vi "MarkedRobot2ndStriker.vi"(6 "atacando ao contrário?":bool=TRUE, 8 "Função":T1, 9 "id":u32, 10 "IA State Input":T3={"our_robots"=[], "enemy_robots"=[], "balls"=[], "geometry"={"line_width"=0, "field_length"=0, "field_width"=0, "boundary_width"=0, "referee_width"=0, "goal_width"=0, "goal_depth"=0, "goal_wall_width"=0, "center_circle_radius"=0, "defense_radius"=0, "defense_stretch"=0, "free_kick_from_defense_dist"=0, "penalty_spot_from_field_line_dist"=0, "penalty_line_from_spot_dist"=0}, "IA Judge"={"stage"="", "command"="", "our_goalie_id"=0.0, "enemy_goalie_id"=0.0, "command enum"=enum."Halt", "Time"=enum."Azul"}, "Received Timestamp"=timestamp(0 s since 1904-01-01), "Events"={"Touch"=FALSE, "Ball out"=FALSE, "id touch"=0.0, "Ball out of \nVision"=FALSE, "Ball inside \nGoalie area"=FALSE, "Robot not responding"=FALSE, "Robots responding status"=[1.0, 1.0, 1.0, 1.0, 1.0, 1.0], "Enemy Ball \nPossession"=FALSE, "Pass State"=FALSE, "id end of pass"=0.0, "Kick"=FALSE, "Id ini Possession"=0.0, "Ball Possesion"=FALSE, "Id Possesion"=0.0, "Direct Kick"=FALSE, "2nd Strk Ativo"=FALSE}}, 11 "AI Parameters":T2={"GotoKick"={"Dist do cone a frente"=150.0, "attacker farback"=1500.0, "Perto"=300.0, "min dist to kick"=150.0, "kick eps"=0.0, "Time to transition"=0.05}, "Attacker"={"CC chute"=0.09, "CC passe"=0.045, "Kick Force"=100.0, "ball-robot Kick"=200.0, "ball-robot Pass"=0.3, "drible\nAttk"=FALSE}, "Defender"={"D max"=1700.0, "Vel p/ robô av"=1000.0, "Kick Force"=100.0, "D atk-def"=0.0, "D farback"=0.0, "drible\ndef"=FALSE, "drible\ngoalie"=FALSE}, "Timeout"={"Field/v in x"=6.0, "Dist Robots"=300, "Dist up in y"=300}, "Pose Striker"={"dist"=200.0, "Numeric"=-4.0, "dist 2"=200.0, "drible\nstriker"=FALSE}, "Dist Stop"=300.0, "D ball out"=200, "D central gap "=150.0, "T pass"=0.0, "Force ++"=0.0, "range kick"=0.0, "Chute alto"=TRUE, "Marcador novo"=TRUE, "drible"=FALSE, "D drible"=300.0, "Versão Striker"=enum."3", "Defesa"=enum."ManMark", "Marcador"=enum."Marcar Segndo mais perigoso", "Receptor passe"=enum."2nd Striker", "Área"=enum."Quadrada"} {"D drible" format="%#_13g"; "D central gap" format="%#_13g"; "Dist Stop" format="%#_13g"; "Pose Striker"."Numeric" format="%#_13g"; "Defender"."Kick Force" format="%#_13g"; "Defender"."Vel p/ robô av" format="%#_13g"; "Attacker"."ball-robot Kick" format="%#_13g"; "Attacker"."Kick Force" format="%#_13g"; "Attacker"."CC passe" format="%#_13g"; "Attacker"."CC chute" format="%#_13g"; "GotoKick"."kick eps" format="%#_13g"; "GotoKick"."min dist to kick" format="%#_13g"; "GotoKick"."Perto" format="%#_13g"; "GotoKick"."attacker farback" format="%#_13g"; "GotoKick"."Dist do cone a frente" format="%#_13g"}) -> (3 "Robô marcado?":bool=TRUE)   [LabVIEW 2017]
uses:
  Core/AI Input.ctl
  Core/AI Robot.ctl
  Functions Enum.ctl
  AttackerStates.ctl
  Path Planning/RRT/PathDests.ctl
  Path Planning/RRT/PathDest.ctl
  Core/AI Ball.ctl
  Core/Field Size.ctl
  Core/AI Judge.ctl
  Command Enum.ctl
  Util/Events/Events.ctl
  AI Parameters.ctl
  d3ae8bea-2540-4cab-b848-3da8b8f91e54.vi
  <vilib>/Array/Sort 2D Array - Pop Stack.vi
  <vilib>/Array/Sort 2D Array - Push Stack.vi
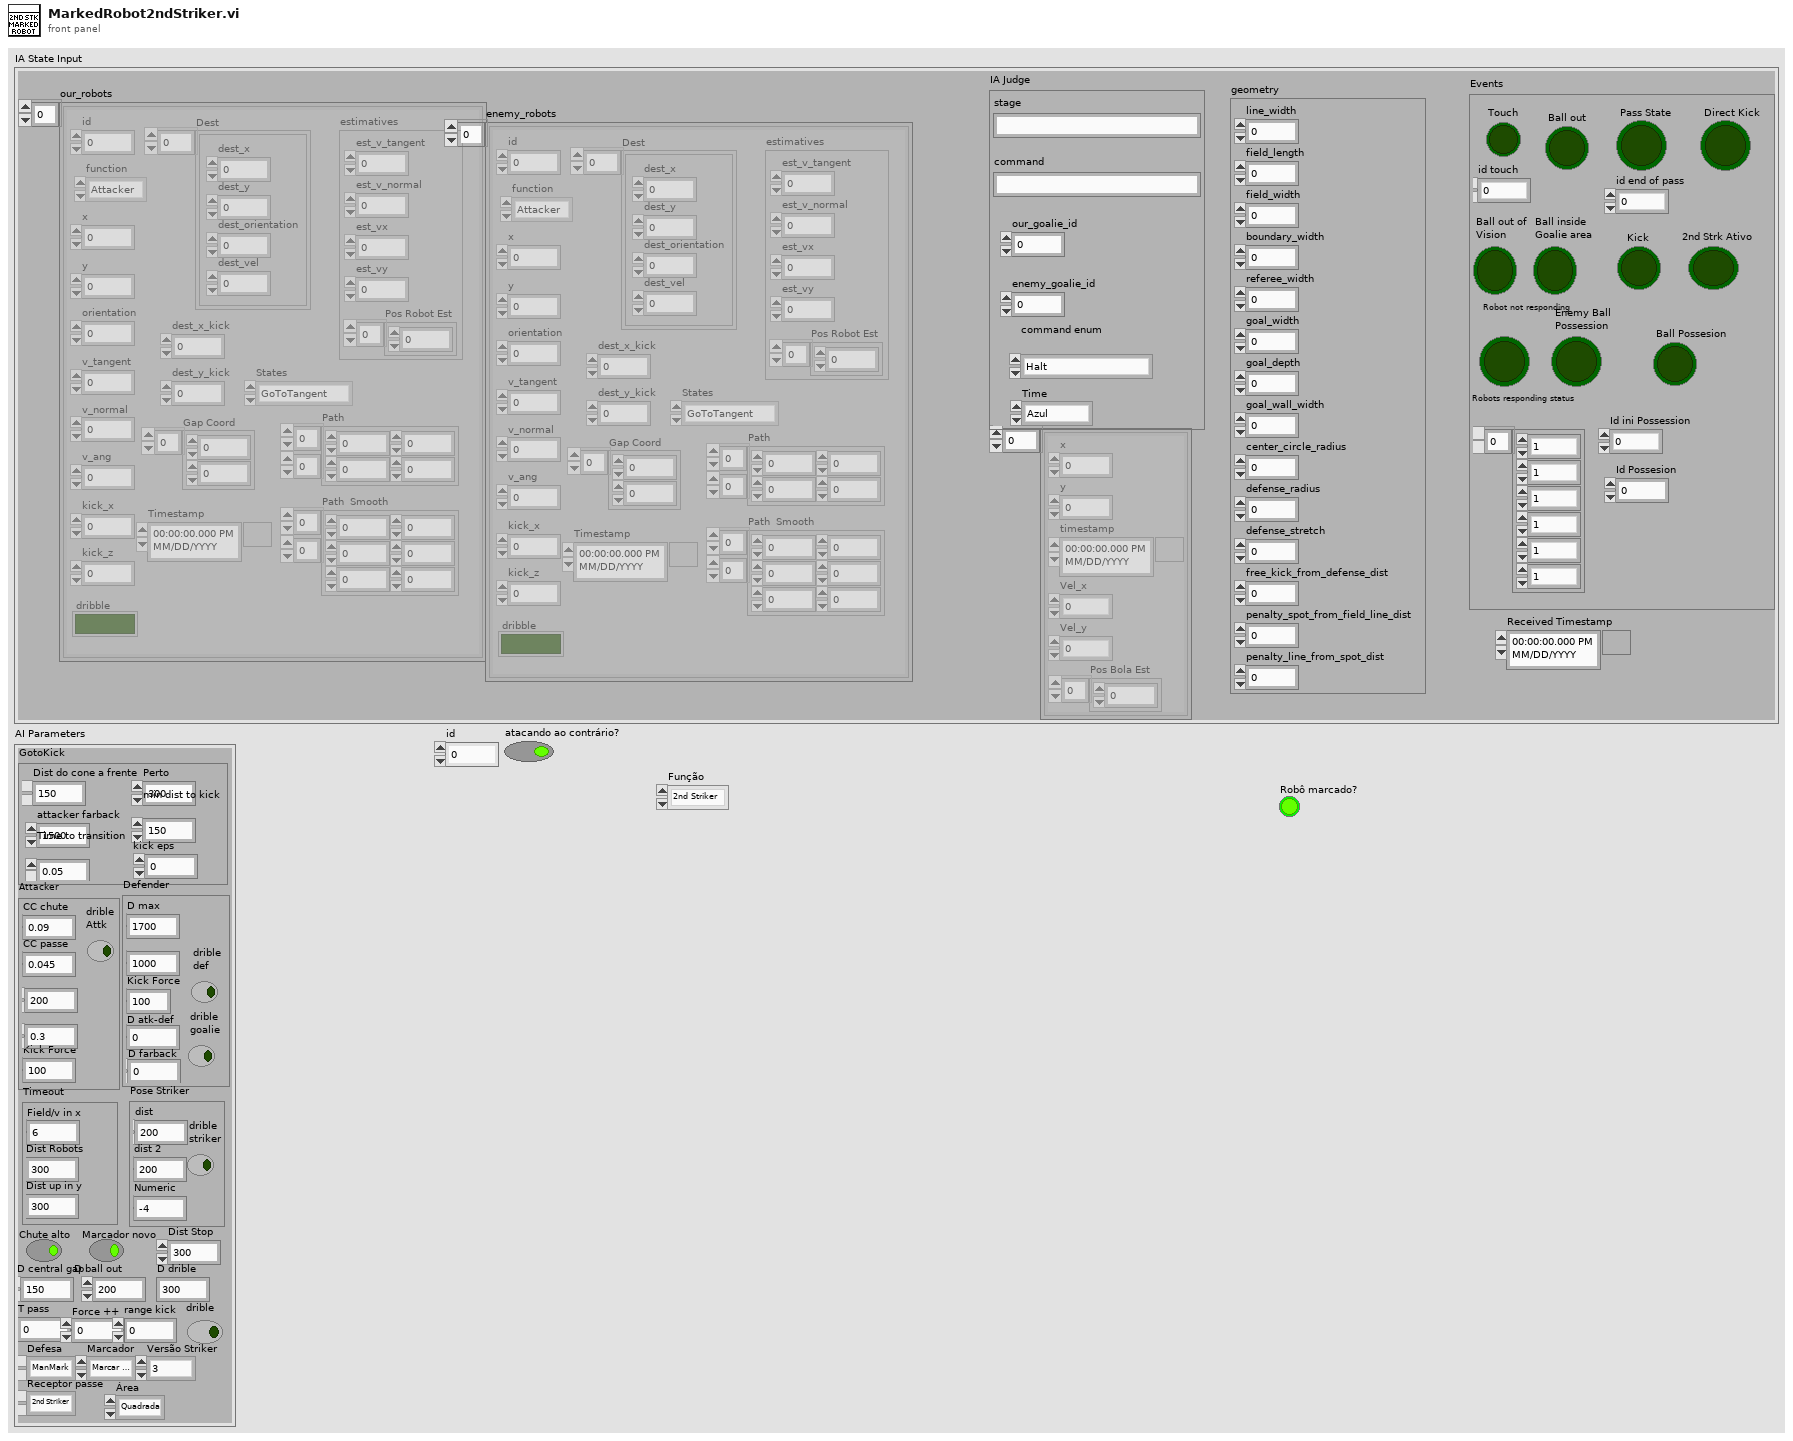
[diagram p1: front panel]
types:
  T1 = typedef "Functions Enum.ctl" = enum16{"2nd Striker", "Attacker", "Goalie", "Defender", "Striker", "Goto 0", "Dummy", "Kicker", "ZigZag 0", "ZigZag 1", "ZigZag 2", "ZigZag 3", "ZigZag 4", "ZigZag 5", "ZigZag 6", "ZigZag 7", "ZigZag 8", ""}
  T2 = typedef "AI Parameters.ctl" = cluster{"GotoKick":cluster{"Dist do cone a frente":dbl, "attacker farback":dbl, "Perto":dbl, "min dist to kick":dbl, "kick eps":dbl, "Time to transition":dbl}, "Attacker":cluster{"CC chute":dbl, "CC passe":dbl, "Kick Force":dbl, "ball-robot Kick":dbl, "ball-robot Pass":dbl, "drible\nAttk":bool}, "Defender":cluster{"D max":dbl, "Vel p/ robô av":dbl, "Kick Force":dbl, "D atk-def":dbl, "D farback":dbl, "drible\ndef":bool, "drible\ngoalie":bool}, "Timeout":cluster{"Field/v in x":dbl, "Dist Robots":u32, "Dist up in y":u32}, "Pose Striker":cluster{"dist":dbl, "Numeric":dbl, "dist 2":dbl, "drible\nstriker":bool}, "Dist Stop":dbl, "D ball out":i32, "D central gap ":dbl, "T pass":dbl, "Force ++":dbl, "range kick":dbl, "Chute alto":bool, "Marcador novo":bool, "drible":bool, "D drible":dbl, "Versão Striker":enum16{"Auto", "3", "2", "1"}, "Defesa":enum16{"ManMark", "Barreira"}, "Marcador":enum16{"Marcar Segndo mais perigoso", "Marcar o mais perigoso"}, "Receptor passe":enum16{"Auto", "2nd Striker", "Striker"}, "Área":enum16{"Quadrada", "Circular"}}
  T3 = typedef "AI Input.ctl" = cluster{"our_robots":T4[], "enemy_robots":T4[], "balls":T8[], "geometry":T9, "IA Judge":T10, "Received Timestamp":timestamp, "Events":T12}
  T4 = typedef "AI Robot.ctl" = cluster{"id":u32, "function":T1, "x":dbl, "y":dbl, "orientation":dbl, "v_tangent":dbl, "v_normal":dbl, "v_ang":dbl, "kick_x":dbl, "kick_z":dbl, "dribble":bool, "Timestamp":timestamp, "estimatives":cluster{"est_v_tangent":dbl, "est_v_normal":dbl, "est_vx":dbl, "est_vy":dbl, "Pos Robot Est":dbl[]}, "dest_x_kick":dbl, "dest_y_kick":dbl, "Gap Coord":dbl[], "States":T5, "Path ":dbl[][], "Path  Smooth":dbl[][], "Dest":T6}
  T5 = typedef "AttackerStates.ctl" = enum16{"Pass", "GoToTangent", "BallGetting", "GoToKick", ""}
  T6 = typedef "PathDests.ctl" = T7[]
  T7 = typedef "PathDest.ctl" = cluster{"dest_x":dbl, "dest_y":dbl, "dest_orientation":dbl, "dest_vel":dbl}
  T8 = typedef "AI Ball.ctl" = cluster{"x":dbl, "y":dbl, "timestamp":timestamp, "Vel_x":dbl, "Vel_y":dbl, "Pos Bola Est":dbl[]}
  T9 = typedef "Field Size.ctl" = cluster{"line_width":u32, "field_length":u32, "field_width":u32, "boundary_width":u32, "referee_width":u32, "goal_width":u32, "goal_depth":u32, "goal_wall_width":u32, "center_circle_radius":u32, "defense_radius":u32, "defense_stretch":u32, "free_kick_from_defense_dist":u32, "penalty_spot_from_field_line_dist":u32, "penalty_line_from_spot_dist":u32}
  T10 = typedef "AI Judge.ctl" = cluster{"stage":string, "command":string, "our_goalie_id":dbl, "enemy_goalie_id":dbl, "command enum":T11, "Time":enum16{"Azul", "Amarelo"}}
  T11 = typedef "Command Enum.ctl" = enum16{"Halt", "Stop", "Force Start", "PKA Normal Start", "Prepare Kickoff Ally", "PKE Normal Start", "Prepare Kickoff Enemy", "Prepare Penalty Ally", "PPA Normal Start", "Prepare Penalty Enemy", "PPE Normal Start", "Direct Free Enemy", "Direct Free Ally", "Indirect Free Enemy", "Indirect Free Ally", "Timeout Enemy", "Timeout Ally", "Goal Enemy", "Goal Ally", "Ball Placement Enemy", "Ball Placement Ally", "Normal Half Time", "Extra Time Break", "Extra Half Time", "None", "Post Game"}
  T12 = typedef "Events.ctl" = cluster{"Touch":bool, "Ball out":bool, "id touch":dbl, "Ball out of \nVision":bool, "Ball inside \nGoalie area":bool, "Robot not responding":bool, "Robots responding status":dbl[], "Enemy Ball \nPossession":bool, "Pass State":bool, "id end of pass":dbl, "Kick":bool, "Id ini Possession":dbl, "Ball Possesion":bool, "Id Possesion":dbl, "Direct Kick":bool, "2nd Strk Ativo":bool}
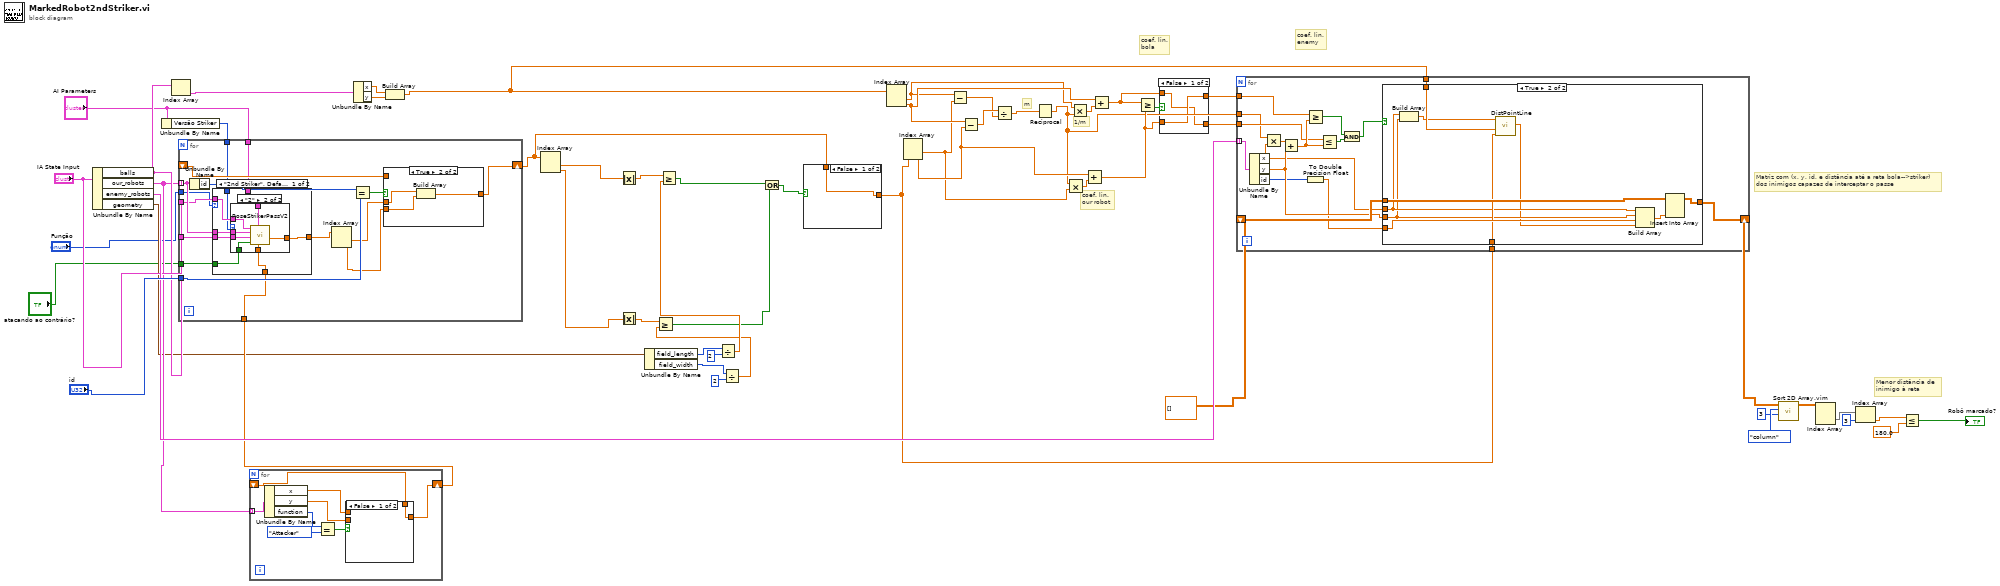
[diagram p0: block diagram]
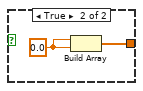
[diagram p2: hidden frame]
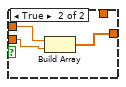
[diagram p3: hidden frame]
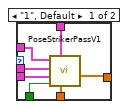
[diagram p6: hidden frame]
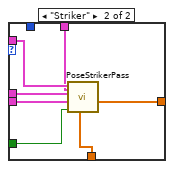
[diagram p7: hidden frame]
diagram:
  # "Menor distância de \ninimigo à reta"
  # "Matriz com (x, y, id, e distância até a reta bola-->striker) \ndos inimigos capazes de interceptar o passe"
  # "coef. lin.\nbola"
  # "coef. lin.\nenemy"
  # "coef. lin.\nour robot"
  # "1/m"
  # "m"
  n1 = Unbundle By Name("IA State Input") -> ("balls"=w28:T8[], "our_robots"=w27:T4[], "enemy_robots"=w46:T4[], "geometry"=w15:T9)
  n2 = Unbundle By Name("AI Parameters") -> ("Versão Striker"=w7:enum16{"Auto", "3", "2", "1"})
  n3 = Index Array(array=w28) -> (element=w54:T8)  [unwired: 1 in]
  n4 = for {
    tunnel: w27 -> [w63] mode=indexing
    shift-right: [w57] -> w26
    shift-left: _ -> [w56]
    n5 = Unbundle By Name(w63) -> ("x"=w59:dbl, "y"=w58:dbl, "function"=w62:T1)
    n6 = Equal?(x=w62, y=Functions_Enum."Attacker") -> (x = y?=w60:bool)
    n7 = case shown="False" w60 {
      tunnel: w59 -> [_ w67]
      tunnel: w58 -> [_ w66]
      tunnel: [w64 w65] -> w57
      tunnel: w56 -> [w64 _]
      frame False {
      }
      frame True {
        n8 = Build Array(w67, w66) -> (w65:dbl[])
      }
    }
  }
  n9 = for {
    tunnel: w27 -> [w75] mode=indexing
    tunnel: "id" -> [w82]
    shift-right: [w80] -> w10
    shift-left: _ -> [w79]
    tunnel: "IA State Input" -> [w74]
    tunnel: w28 -> [w73]
    tunnel: "AI Parameters" -> [w72]
    tunnel: w26 -> [w71]
    tunnel: "Função" -> [w70]
    tunnel: w7 -> [w69]
    tunnel: "atacando ao contrário?" -> [w68]
    n10 = Unbundle By Name(w75) -> ("id"=w83:u32)
    n11 = case shown="\"2nd Striker\", Default" w70 {
      tunnel: [w91 w112] -> w78
      tunnel: w75 -> [w88 w111]
      tunnel: w74 -> [w89 w110]
      tunnel: w73 -> [w87 w109]
      tunnel: w72 -> [w90 w108]
      tunnel: w71 -> [w86 w107]
      tunnel: w69 -> [w85 _]
      tunnel: w68 -> [w84 w106]
      frame "2nd Striker", Default {
        n12 = case shown="\"2\"" w85 {
          tunnel: [w97 w105] -> w91
          tunnel: w90 -> [w94 w104]
          tunnel: w89 -> [w93 w103]
          tunnel: w88 -> [w95 w102]
          tunnel: w87 -> [w96 w101]
          tunnel: w86 -> [w98 w100]
          tunnel: w84 -> [w92 w99]
          frame "1", Default {
            n13 = call "PoseStrikerPassV1.vi"("Array"=w98, "AI Parameters"=w94, "atacando ao contrário?"=w92, "balls"=w96, "Robot in"=w95, "IA Input"=w93) -> ("FinalPosition"=w97:dbl[])  [unwired: 4 in, 1 out]
          }
          frame "2" {
            n14 = call "PoseStrikerPassV2.vi"("Array"=w100, "AI Parameters"=w104, "atacando ao contrário?"=w99, "balls"=w101, "Robot in"=w102, "IA Input"=w103) -> ("FinalPosition"=w105:dbl[])  [unwired: 4 in, 1 out]
          }
        }
      }
      frame "Striker" {
        n15 = call "PoseStrikerPass.vi"("Array"=w107, "AI Parameters"=w108, "atacando ao contrário?"=w106, "balls"=w109, "Robot in"=w111, "IA Input"=w110) -> ("FinalPosition"=w112:dbl[])  [unwired: 4 in, 1 out]
      }
    }
    n16 = Index Array(array=w78) -> (element #1=w77:dbl, element #2=w76:dbl)  [unwired: 2 in]
    n17 = Equal?(x=w83, y=w82) -> (x = y?=w81:bool)
    n18 = case shown="True" w81 {
      tunnel: w77 -> [_ w116]
      tunnel: w76 -> [_ w115]
      tunnel: [w113 w114] -> w80
      tunnel: w79 -> [w113 _]
      frame False {
      }
      frame True {
        n19 = Build Array(w116, w115) -> (w114:dbl[])
      }
    }
  }
  n20 = Unbundle By Name(w54) -> ("x"=w53:dbl, "y"=w52:dbl)
  n21 = Build Array(w53, w52) -> (w39:dbl[])
  n22 = Index Array(array=w10) -> (element #1=w14:dbl, element #2=w13:dbl)  [unwired: 2 in]
  n23 = Absolute Value(x=w14) -> (abs(x)=w21:dbl)
  n24 = Absolute Value(x=w13) -> (abs(x)=w19:dbl)
  n25 = Unbundle By Name(w15) -> ("field_length"=w25:u32, "field_width"=w22:u32)
  n26 = Divide(x=w25, y=2) -> (x/y=w20:dbl)
  n27 = Greater Or Equal?(x=w21, y=w20) -> (x >= y?=w17:bool)
  n28 = Divide(x=w22, y=u32 2) -> (x/y=w18:dbl)
  n29 = Greater Or Equal?(x=w19, y=w18) -> (x >= y?=w16:bool)
  n30 = Or(x=w17, y=w16) -> (x .or. y?=w12:bool)
  n31 = case shown="False" w12 {
    tunnel: [w117 w118] -> w11
    tunnel: w10 -> [w117 _]
    frame False {
    }
    frame True {
      w119 = 0.0
      n32 = Build Array(w119, w119) -> (w118:dbl[])
    }
  }
  n33 = Index Array(array=w39) -> (element #1=w3:dbl, element #2=w50:dbl)  [unwired: 2 in]
  n34 = Index Array(array=w11) -> (element #1=w4:dbl, element #2=w49:dbl)  [unwired: 2 in]
  n35 = Subtract(x=w3, y=w4) -> (x-y=w47:dbl)
  n36 = Subtract(x=w50, y=w49) -> (x-y=w48:dbl)
  n37 = Divide(x=w48, y=w47) -> (x/y=w51:dbl)
  n38 = Reciprocal(x=w51) -> (1/x=w1:dbl)
  n39 = Multiply(x=w1, y=w4) -> (x*y=w5:dbl)
  n40 = Multiply(x=w3, y=w1) -> (x*y=w2:dbl)
  n41 = Add(x=w49, y=w5) -> (x+y=w43:dbl)
  n42 = Add(x=w50, y=w2) -> (x+y=w44:dbl)
  n43 = Greater Or Equal?(x=w44, y=w43) -> (x >= y?=w45:bool)
  n44 = case shown="False" w45 {
    tunnel: [w121 w123] -> w42
    tunnel: w44 -> [w120 w123]
    tunnel: [w120 w122] -> w41
    tunnel: w43 -> [w121 w122]
    frame False {
    }
    frame True {
    }
  }
  n45 = for {
    tunnel: w46 -> [w140] mode=indexing
    tunnel: w1 -> [w124]
    shift-right: [w138] -> w37
    shift-left: dbl[][] [] -> [w139]
    tunnel: w42 -> [w133]
    tunnel: w41 -> [w132]
    tunnel: w39 -> [w128]
    tunnel: w11 -> [w127]
    n46 = Unbundle By Name(w140) -> ("x"=w126:dbl, "y"=w131:dbl, "id"=w130:u32)
    n47 = Multiply(x=w124, y=w126) -> (x*y=w125:dbl)
    n48 = Add(x=w125, y=w131) -> (x+y=w137:dbl)
    n49 = Greater Or Equal?(x=w133, y=w137) -> (x >= y?=w135:bool)
    n50 = To Double Precision Float(number=w130) -> (double precision float=w129:dbl)
    n51 = Less Or Equal?(x=w132, y=w137) -> (x <= y?=w136:bool)
    n52 = And(x=w135, y=w136) -> (x .and. y?=w134:bool)
    n53 = case shown="True" w134 {
      tunnel: w139 -> [w141 w151]
      tunnel: [w141 w150] -> w138
      tunnel: w126 -> [_ w145]
      tunnel: w131 -> [_ w144]
      tunnel: w129 -> [_ w149]
      tunnel: w128 -> [_ w147]
      tunnel: w127 -> [_ w146]
      frame False {
      }
      frame True {
        n54 = Build Array(w145, w144) -> (w143:dbl[])
        n55 = call "DistPointLine.vi"("P2"=w146, "P1"=w147, "Q"=w143) -> ("distance"=w142:dbl)  [unwired: 8 in]
        n56 = Build Array(w145, w144, w149, w142) -> (w148:dbl[])
        n57 = Insert Into Array(array=w151, new element=w148) -> (w150:dbl[][])  [unwired: 2 in]
      }
    }
  }
  n58 = call "Sort 2D Array.vim"("index"=3, "dimension to index (column)"=enum16{"column", "row"}."column", "2D array"=w37) -> ("sorted 2D array"=w36:dbl[][])  [unwired: 7 in, 1 out]
  n59 = Index Array(array=w36) -> (element=w35:dbl[])  [unwired: 2 in]
  n60 = Index Array(array=w35, index=3) -> (element=w32:dbl)
  n61 = Less Or Equal?(x=w32, y=180.0) -> (x <= y?=→"Robô marcado?":bool)
